vi "AO_single_Host.vi"() -> ()   [LabVIEW 2021]
uses:
  <vilib>/rvi/Analysis/host/Private/Sample Rate To Loop Time (ticks).vi
  <vilib>/FPGAPlugInAG/PCIe-7857/niLvFpga_Open_PCIe-7857.vi
  <vilib>/rvi/interface/common/dynamic/niFpgaDynamicAddResources.vi
  <vilib>/Utility/error.llb/Error Cluster From Error Code.vi
  <vilib>/rvi/errors/niLvFpgaAdjustHostInterfaceError.vi
  <vilib>/rvi/interface/common/niFpgaWaitOnOcc.vi
  <vilib>/FPGAPlugInAG/Dynamic/niLvFpga_Run_Dynamic.vi
  <vilib>/FPGAPlugInAG/Dynamic/niLvFpga_Close_Dynamic.vi
  <vilib>/rvi/interface/nirviOpenFPGA/nirviOpenFPGA.xnode
  FPGA Bitfiles/lvfpga2_FPGATarget_AOsingleFPGA_2V+HchRLk9w.lvbitx
  AO_single_FPGA.vi
  <vilib>/rvi/interface/nirviReadWriteControl/nirviReadWriteControl.xnode
  <vilib>/rvi/interface/nirviMethod/nirviMethod.xnode
  <vilib>/rvi/interface/nirviCloseFPGA/nirviCloseFPGA.xnode
  <vilib>/rvi/interface/Simulation/niFpgaSimulationCallBeginRW.vi
  <vilib>/rvi/Analysis/host/Public/NI_FpgaMspHost.lvlib
  <vilib>/rvi/errors/niLvFpgaMergeErrorWithErrorCode.vi
  <vilib>/FPGAPlugInAG/Dynamic/niLvFpga_WriteFifo_Dynamic.vi
  NiFpgaLv.dll
  <vilib>/FPGAPlugInAG/Dynamic/niLvFpga_ConfigureFifo_Dynamic.vi
panel:
  out "Actual #s":dbl
  in  "stop":bool
  out "Actual Sample Clock Rate":dbl=20000.0 format="%.2f"
  out "Waveform Graph":waveform(dbl)(graph)
  in  "scale":sgl=1.0 format="%0.2f"
  in  "offset":sgl format="%0.2p"
  in  "functionInfo":T1={"time1"=5e-05, "formula1"="2", "time2"=5e-05, "formula2"="3", "time3"=0.0005, "formula3"="4", "time4"=0.001, "formula4"="1"}
  out "Actual Depth":u32
  in  "Signal Parameters":cluster{"Fs":dbl, "#s":dbl}={"Fs"=200000.0, "#s"=100.0} {"Fs" format="%#_6p"}
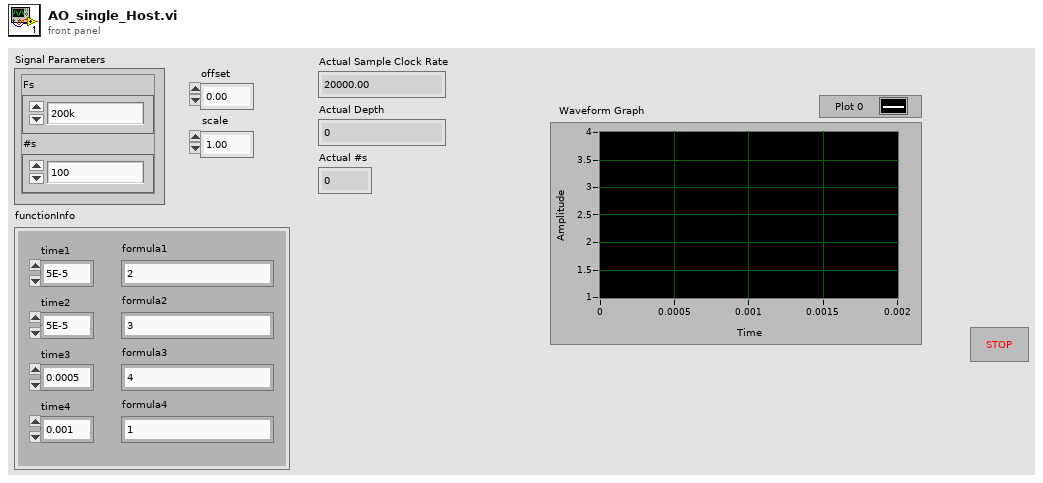
[diagram p1: front panel]
types:
  T1 = cluster{"time1":dbl, "formula1":string, "time2":dbl, "formula2":string, "time3":dbl, "formula3":string, "time4":dbl, "formula4":string}
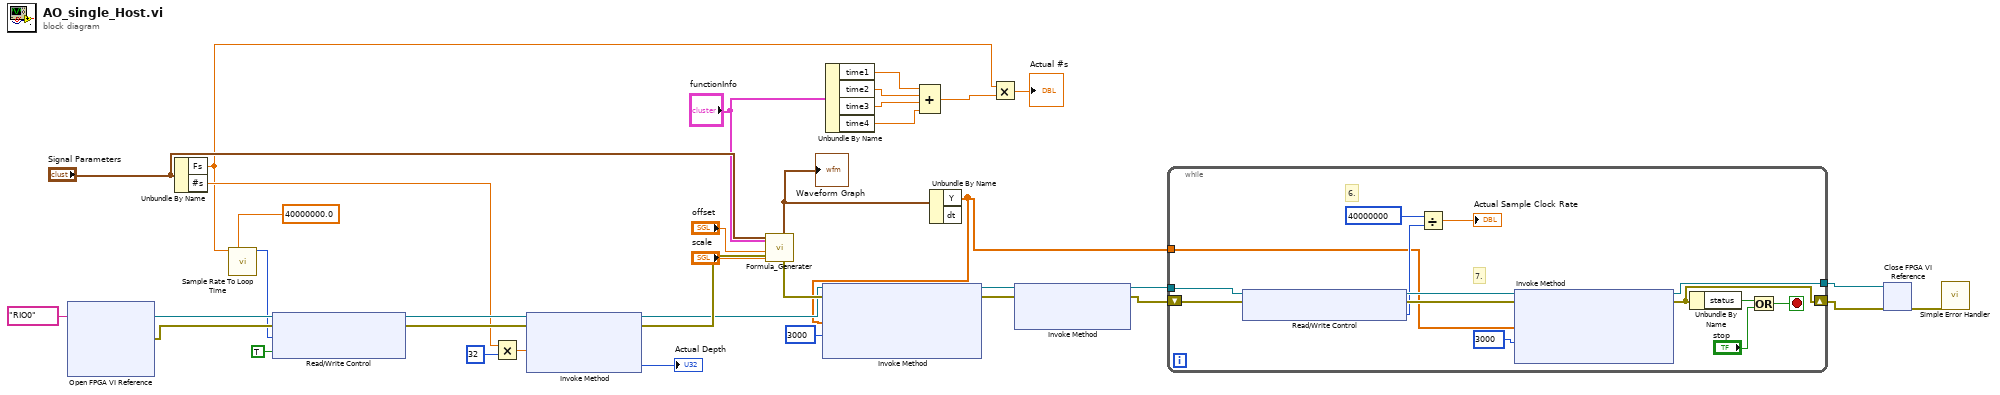
[diagram p0: block diagram]
diagram:
  n1 = xnode "Open FPGA VI Reference"("resource name"=tag "RIO0") -> ("FPGA VI Reference Out"=w35:refnum<k20>, "error out"=w34:errorcluster)  [unwired: 1 in]
  n2 = Unbundle By Name("Signal Parameters") -> ("Fs"=w2:dbl, "#s"=w25:dbl)
  n3 = call-poly <vilib>:"Sample Rate To Loop Time.vi"("sample rate (S/s)"=w2, "FPGA clock rate (Hz)"=40000000.0) -> ("count (ticks/S)"=w32:u32)  [unwired: 11 in, 2 out]
  n4 = xnode "Read/Write Control"("FPGA VI Reference In"=w35, "error in"=w34, "AO Loop Timer (ticks)"=w32, "AO Enable"=TRUE) -> ("FPGA VI Reference Out"=w27:refnum<k20>, "error out"=w26:errorcluster)
  n5 = Multiply(x=w25, y=u32 32) -> (x*y=w29:dbl)
  n6 = xnode "Invoke Method"("FPGA VI Reference In"=w27, "error in"=w26, "Requested Depth"=w29) -> ("FPGA VI Reference Out"=w18:refnum<k20>, "error out"=w21:errorcluster, "Actual Depth"=→"Actual Depth":u32)
  n7 = call "Formula_Generater.vi"("error in (no error)"=w21, "functionInfo"="functionInfo", "scale"="scale", "offset"="offset", "sampling info"="Signal Parameters") -> ("error out"=w20:errorcluster, "waveform out"=w13:waveform(dbl))  [unwired: 5 in]
  "Waveform Graph" <- w13
  n8 = Unbundle By Name("functionInfo") -> ("time1"=w9:dbl, "time2"=w8:dbl, "time3"=w7:dbl, "time4"=w6:dbl)
  n9 = Compound Arithmetic op=ADD(w9, w8, w7, w6) -> (w5:dbl)
  n10 = Unbundle By Name(w13) -> ("Y"=w1:dbl[])  [unwired: 1 out]
  n11 = xnode "Invoke Method"("FPGA VI Reference In"=w18, "error in"=w20, "Data"=w1, "Timeout (ms)"=3000) -> ("FPGA VI Reference Out"=w17:refnum<k20>, "error out"=w16:errorcluster)  [unwired: 1 out]
  n12 = Multiply(x=w2, y=w5) -> (x*y=→"Actual #s":dbl)
  n13 = xnode "Invoke Method"("FPGA VI Reference In"=w17, "error in"=w16) -> ("FPGA VI Reference Out"=w14:refnum<k20>, "error out"=w15:errorcluster)  [unwired: 1 in]
  n14 = while {
    tunnel: w14 -> [w48]
    shift-right: [w40] -> w11
    shift-left: w15 -> [w37]
    tunnel: [w50] -> w12
    tunnel: w1 -> [w38]
    stop <- w41 stop-if-true
    # "7."
    # "6."
    n15 = xnode "Read/Write Control"("FPGA VI Reference In"=w48, "error in"=w37) -> ("FPGA VI Reference Out"=w47:refnum<k20>, "error out"=w46:errorcluster, "AO: Actual Loop Rate (ticks)"=w45:u32)
    n16 = Divide(x=u32 40000000, y=w45) -> (x/y=→"Actual Sample Clock Rate":dbl)
    n17 = xnode "Invoke Method"("FPGA VI Reference In"=w47, "error in"=w46, "Data"=w38, "Timeout (ms)"=3000) -> ("FPGA VI Reference Out"=w50:refnum<k20>, "error out"=w40:errorcluster)  [unwired: 1 out]
    n18 = Unbundle By Name(w40) -> ("status"=w39:bool)
    n19 = Or(x=w39, y="stop") -> (x .or. y?=w41:bool)
  }
  n20 = xnode "Close FPGA VI Reference"("FPGA VI Reference In"=w12, "error in"=w11) -> ("error out"=w10:errorcluster)
  n21 = call <vilib>:"Simple Error Handler.vi"("error in (no error)"=w10) -> ()  [unwired: 4 in, 5 out]
